vi "BackEnd_Module.vi"() -> ()   [LabVIEW 2023]
uses:
  Controls/Quantity_Data.ctl
  Controls/Queue_Operation_Select.ctl
  Controls/State_and_Data.ctl
  Controls/File_Operation_Select.ctl
panel:
  in  "Error_In":errorcluster
  out "error constant":errorcluster
  in  "Backend_Data":T1 {"Level"."Milk_Level" scale=0.0..100.0; "Level"."Bean_Level" scale=0.0..100.0; "Level"."Water_Level" scale=0.0..100.0}
  # "COFFEE MACHINE"
  # "Backend Control Panel"
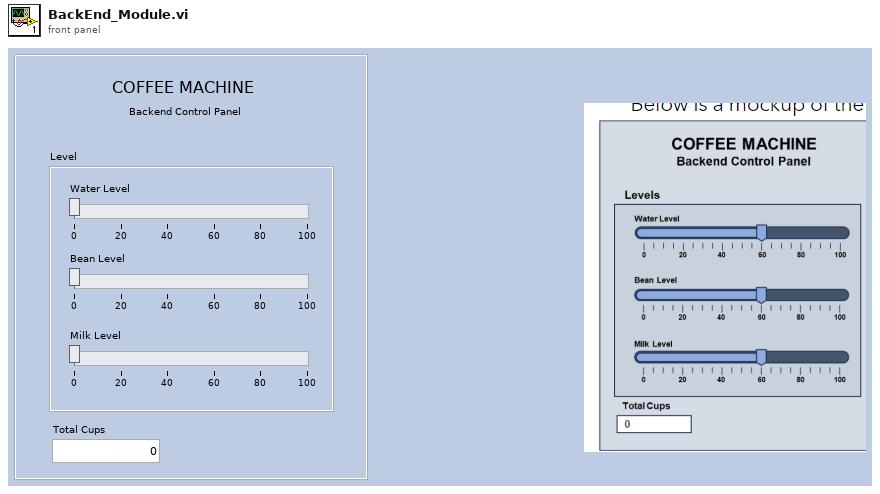
[diagram p1: front panel]
types:
  T1 = typedef "Quantity_Data.ctl" = cluster{"Level":cluster{"Water_Level":dbl, "Bean_Level":dbl, "Milk_Level":dbl}, "Total_Cups":dbl}
  T2 = typedef "File_Operation_Select.ctl" = enum16{"Open", "Read", "Write", "Close"}
  T3 = typedef "State_and_Data.ctl" = cluster{"State":string, "Data":variant}
  T4 = typedef "Queue_Operation_Select.ctl" = enum16{"Obtain_Queue", "Enqueue", "Enqueue_First", "Enqueue_N", "Lossy_Enqueue", "Preview", "Queue_Status", "Dequeue", "Flush", "Release_Queue"}
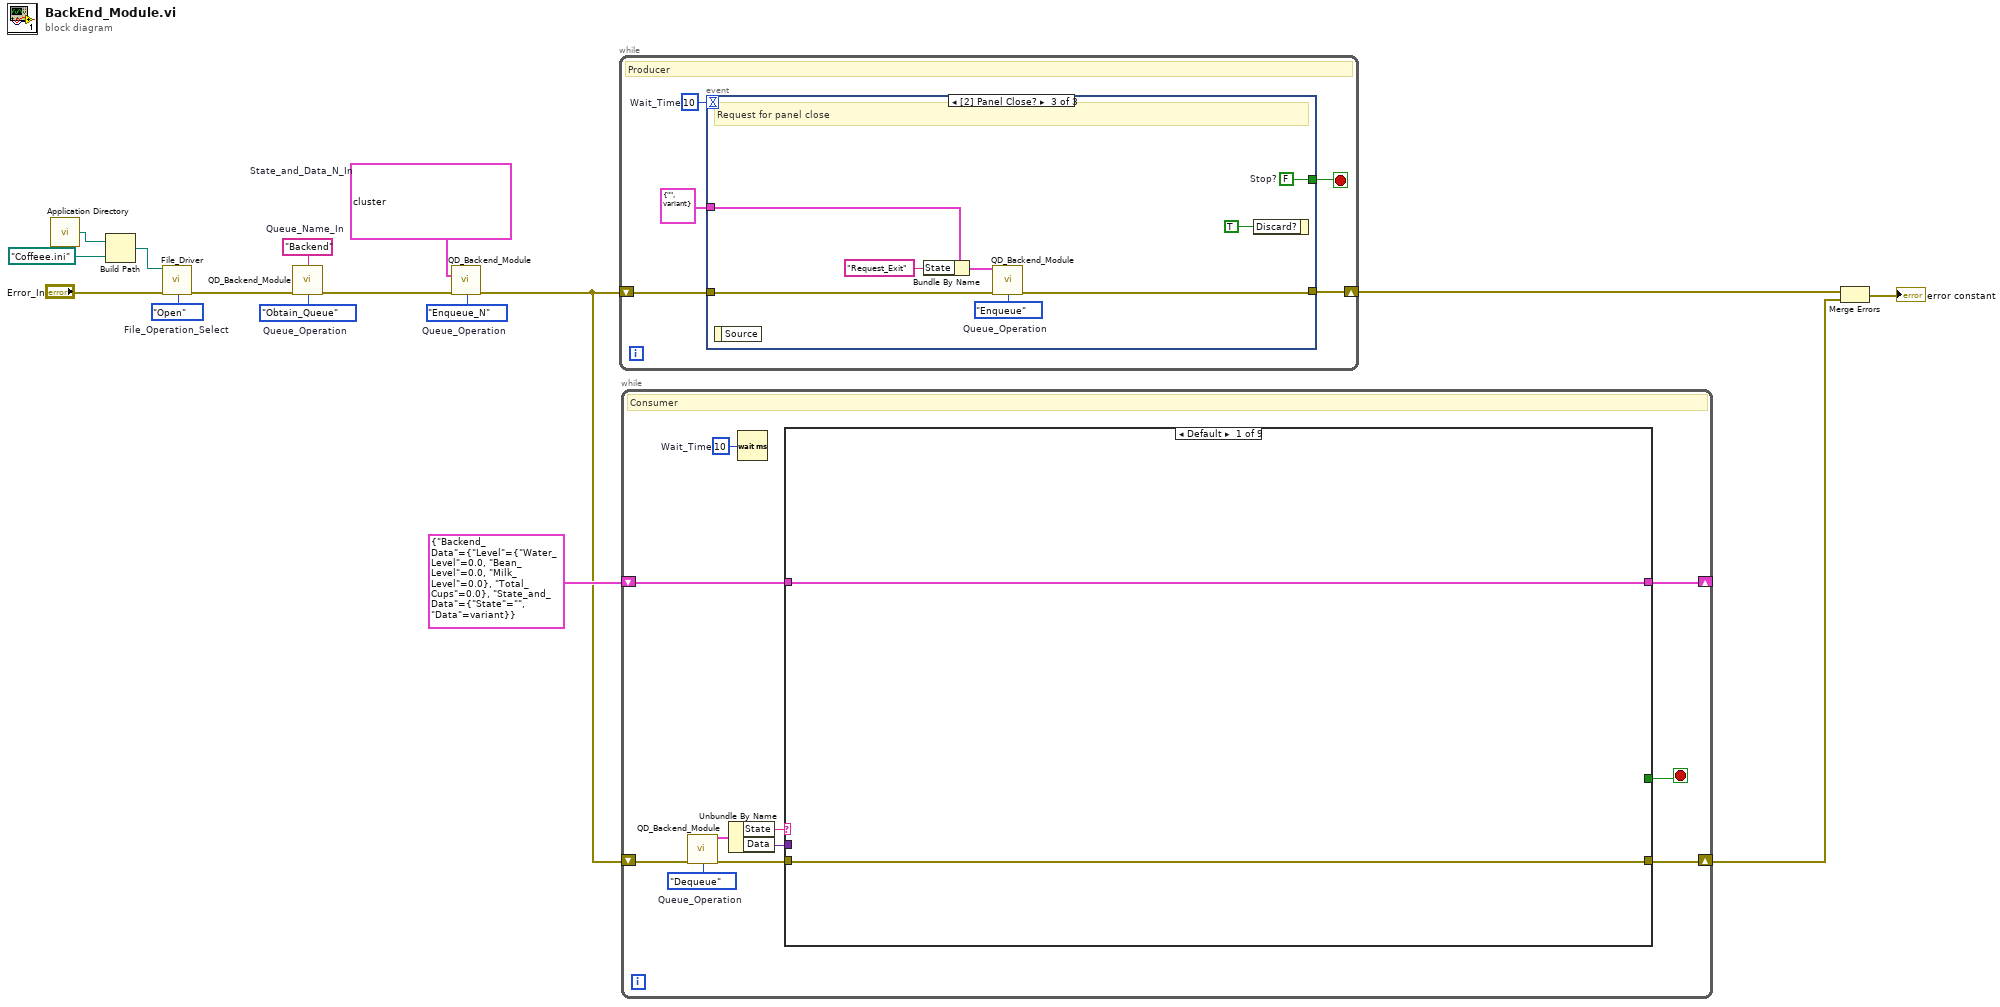
[diagram p0: block diagram]
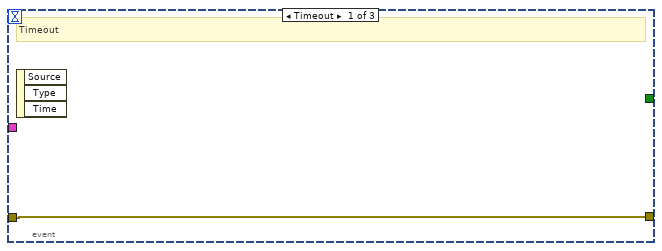
[diagram p2: hidden frame]
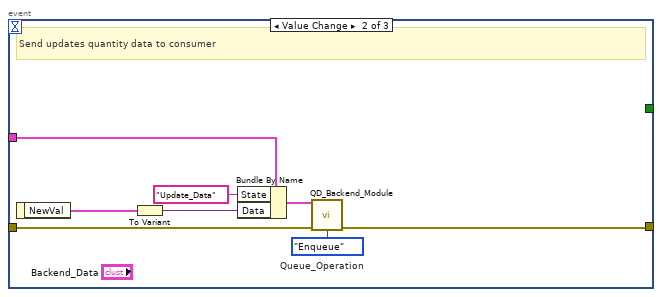
[diagram p3: hidden frame]
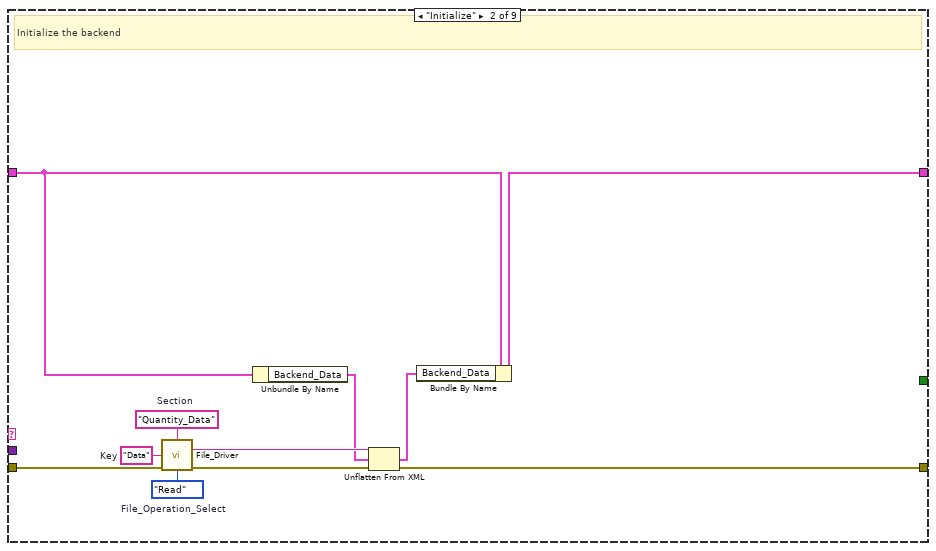
[diagram p4: hidden frame]
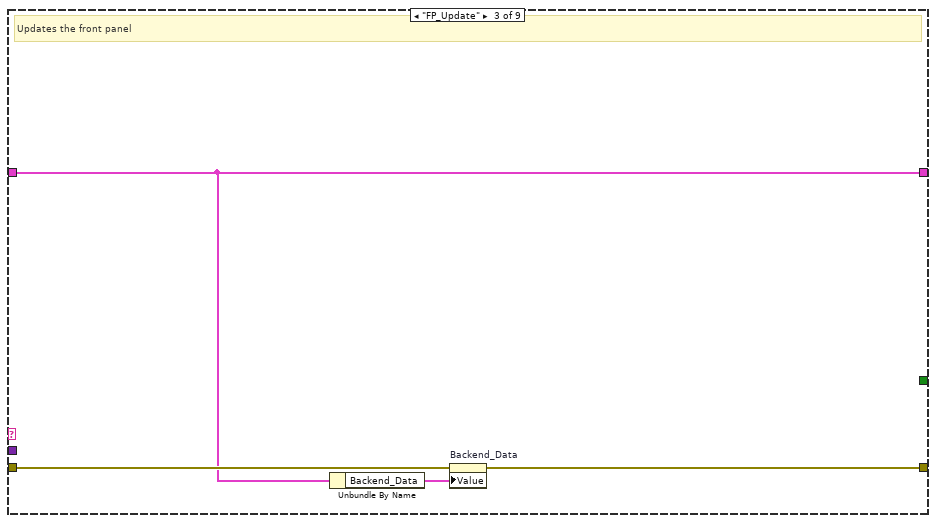
[diagram p5: hidden frame]
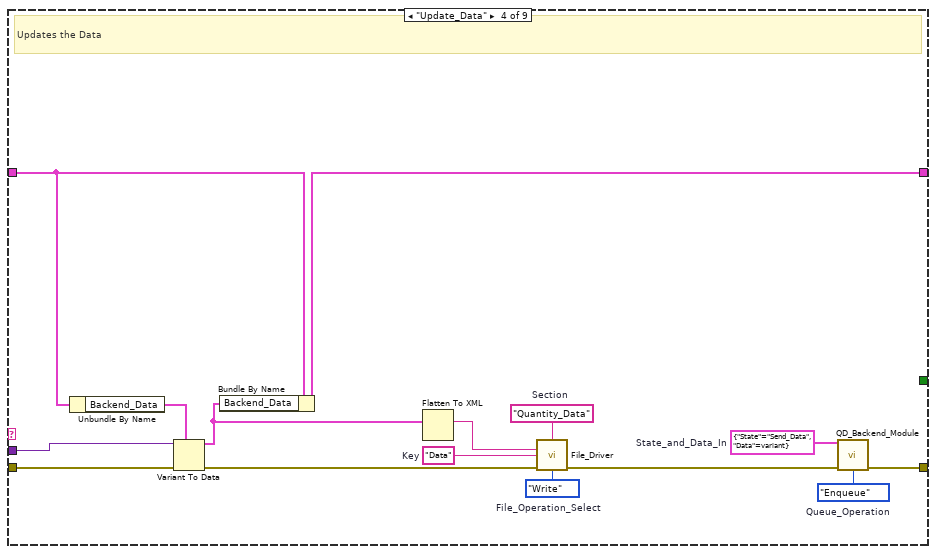
[diagram p6: hidden frame]
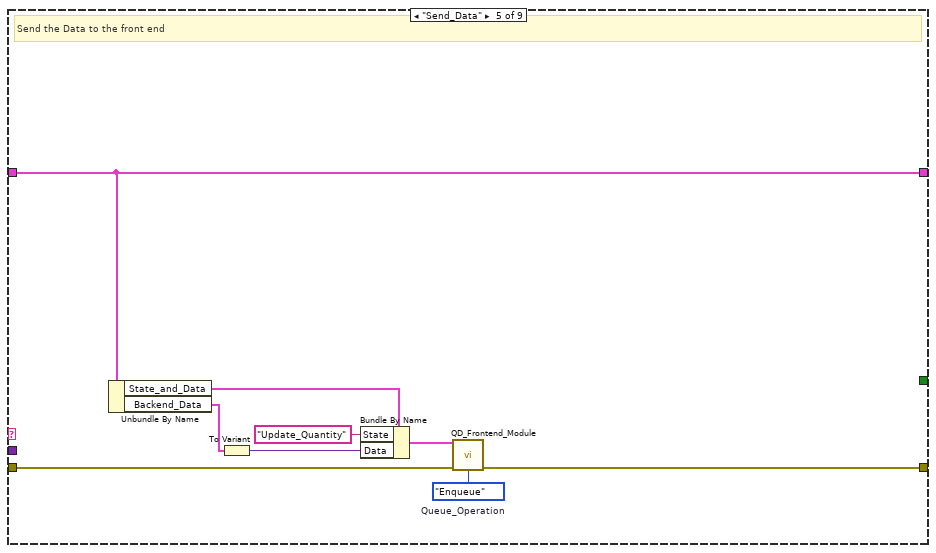
[diagram p7: hidden frame]
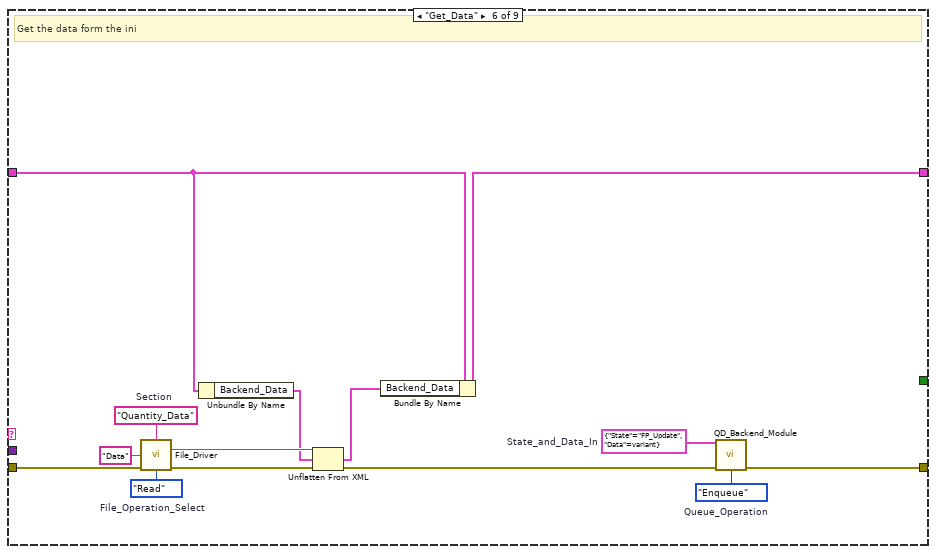
[diagram p8: hidden frame]
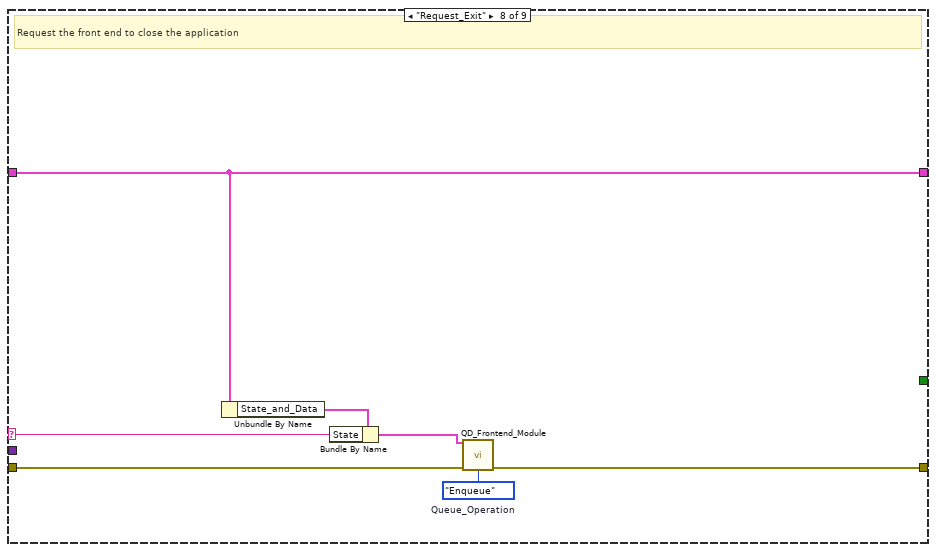
[diagram p10: hidden frame]
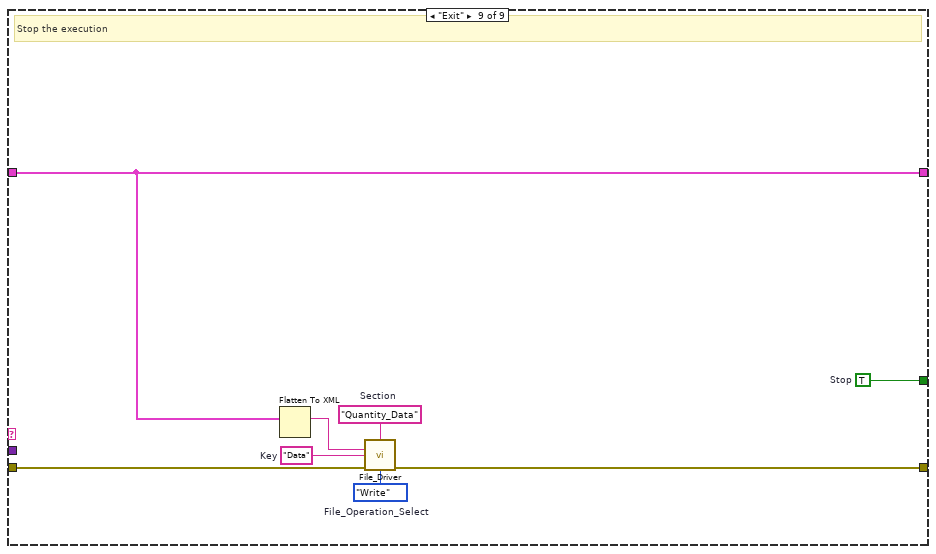
[diagram p11: hidden frame]
diagram:
  w5 = File_Operation_Select."Open"  # File_Operation_Select
  w10 = T3[] [{"State"="Initialize", "Data"=variant(cluster{"Current_Data":dbl, "Temp_Data":dbl} {"Current_Data"=0.0, "Temp_Data"=0.0})}, {"State"="FP_Update", "Data"=variant(cluster{"Current_Data":dbl, "Temp_Data":dbl} {"Current_Data"=0.0, "Temp_Data"=0.0})}]  # State_and_Data_N_In
  w11 = Queue_Operation_Select."Enqueue_N"  # Queue_Operation
  w12 = "Backend"  # Queue_Name_In
  w13 = Queue_Operation_Select."Obtain_Queue"  # Queue_Operation
  n1 = call <vilib>:"Application Directory.vi"() -> ("Application Directory"=w9:path)
  n2 = Build Path(base path=w9, name or relative path=path "Coffeee.ini") -> (appended path=w4:path)
  n3 = call "File_Driver.vi"("File_Path"=w4, "Error_In"="Error_In", "File_Operation_Select"=w5) -> ("Error_Out"=w6:errorcluster)  [unwired: 11 in, 1 out]
  n4 = call "QD_Backend_Module.vi"("Queue_Name_In"=w12, "Error_In"=w6, "Queue_Operation"=w13) -> ("Error_Out"=w14:errorcluster)  [unwired: 10 in, 2 out]
  n5 = call "QD_Backend_Module.vi"("State_and_Data_N_In"=w10, "Error_In"=w14, "Queue_Operation"=w11) -> ("Error_Out"=w1:errorcluster)  [unwired: 10 in, 2 out]
  n6 = while {
    shift-right: [w21] -> w16
    shift-left: w1 -> [w20]
    stop <- w19 stop-if-true
    w17 = 10  # Wait_Time
    # "Producer"
    n7 = event shown="[2] Panel Close?" {
      selector: _ -> [_ _ _]
      dyn-events: _ -> [_ _ _]
      timeout: w17 -> [_ _ _]
      tunnel: [w22 w29 w37] -> w21
      tunnel: w20 -> [w22 w30 w38]
      tunnel: [_ _ w34] -> w19
      tunnel: T3 {"State"="", "Data"=variant} ("State_and_Data_In") -> [_ w24 w32]
      event Timeout {
        # "Timeout"
        n8 = event-data() -> ()  [unwired: 1 in, 3 out]
      }
      event Value Change {
        w28 = Queue_Operation_Select."Enqueue"  # Queue_Operation
        # "Send updates quantity data to consumer"
        n9 = event-data() -> ("NewVal"=w26:T1)  [unwired: 1 in]
        n10 = To Variant(anything=w26) -> (Variant=w25:variant)
        n11 = Bundle By Name(cluster=w24, "State"="Update_Data", "Data"=w25) -> (w27:T3)
        n12 = call "QD_Backend_Module.vi"("State_and_Data_In"=w27, "Error_In"=w30, "Queue_Operation"=w28) -> ("Error_Out"=w29:errorcluster)  [unwired: 10 in, 2 out]
      }
      event Panel Close? {
        w34 = FALSE  # Stop?
        w36 = Queue_Operation_Select."Enqueue"  # Queue_Operation
        # "Request for panel close"
        n13 = event-data() -> ()  [unwired: 1 in, 1 out]
        n14 = Bundle By Name(cluster=w32, "State"="Request_Exit") -> (w35:T3)
        n15 = call "QD_Backend_Module.vi"("State_and_Data_In"=w35, "Error_In"=w38, "Queue_Operation"=w36) -> ("Error_Out"=w37:errorcluster)  [unwired: 10 in, 2 out]
        n16 = event-data("Discard?"=TRUE) -> ()  [unwired: 1 in, 1 out]
      }
    }
  }
  n17 = while {
    shift-right: [w49] -> w2
    shift-left: w1 -> [w48]
    shift-right: [w43] -> _
    shift-left: cluster{"Backend_Data":T1, "State_and_Data":T3} {"Backend_Data"={"Level"={"Water_Level"=0.0, "Bean_Level"=0.0, "Milk_Level"=0.0}, "Total_Cups"=0.0}, "State_and_Data"={"State"="", "Data"=variant}} -> [w42]
    stop <- w41 stop-if-true
    w40 = u32 10  # Wait_Time
    w46 = Queue_Operation_Select."Dequeue"  # Queue_Operation
    # "Consumer"
    n18 = call "QD_Backend_Module.vi"("Error_In"=w48, "Queue_Operation"=w46) -> ("State_and_Data_Out"=w39:T3, "Error_Out"=w47:errorcluster)  [unwired: 11 in, 1 out]
    n19 = Unbundle By Name(w39) -> ("State"=w45:string, "Data"=w44:variant)
    n20 = Wait (ms)(milliseconds to wait=w40) -> ()  [unwired: 1 out]
    n21 = case shown="Default" w45 {
      selector: w45 -> [_ _ _ _ _ _ _ w108 _]
      tunnel: [w51 w52 w65 w69 w89 w103 w106 w112 w120] -> w49
      tunnel: w47 -> [w51 w62 w66 w81 w90 w100 w106 w113 w121]
      tunnel: w44 -> [_ _ _ w78 _ _ _ _ _]
      tunnel: [w50 w54 w64 w80 w88 w104 w105 w110 w116] -> w43
      tunnel: w42 -> [w50 w56 w64 w77 w88 w92 w105 w110 w116]
      tunnel: [_ _ _ _ _ _ _ _ w114] -> w41
      frame Default {
      }
      frame "Initialize" {
        w58 = "Data"  # Key
        w59 = "Quantity_Data"  # Section
        w60 = File_Operation_Select."Read"  # File_Operation_Select
        # "Initialize the backend"
        n22 = call "File_Driver.vi"("Section"=w59, "Key"=w58, "Error_In"=w62, "File_Operation_Select"=w60) -> ("Data_Out"=w57:string, "Error_Out"=w61:errorcluster)  [unwired: 10 in]
        n23 = Unbundle By Name(w56) -> ("Backend_Data"=w55:T1)
        n24 = Unflatten From XML(xml string=w57, type=w55, error in (no error)=w61) -> (value=w53:T1, error out=w52:errorcluster)
        n25 = Bundle By Name(cluster=w56, "Backend_Data"=w53) -> (w54:cluster{"Backend_Data":T1, "State_and_Data":T3})
      }
      frame "FP_Update" {
        # "Updates the front panel"
        n26 = Unbundle By Name(w64) -> ("Backend_Data"=w63:T1)
        n27 = property on="Backend_Data" class="Clust (strict)"(error in=w66, "Value"=w63) -> (error out=w65:errorcluster)  [unwired: 1 in, 1 out]
      }
      frame "Update_Data" {
        w67 = Queue_Operation_Select."Enqueue"  # Queue_Operation
        w68 = T3 {"State"="Send_Data", "Data"=variant}  # State_and_Data_In
        w72 = "Quantity_Data"  # Section
        w73 = "Data"  # Key
        w74 = File_Operation_Select."Write"  # File_Operation_Select
        # "Updates the Data"
        n28 = Unbundle By Name(w77) -> ("Backend_Data"=w76:T1)
        n29 = Variant To Data(error in=w81, type=w76, Variant=w78) -> (data=w71:T1, error out=w79:errorcluster)
        n30 = Bundle By Name(cluster=w77, "Backend_Data"=w71) -> (w80:cluster{"Backend_Data":T1, "State_and_Data":T3})
        n31 = Flatten To XML(6:w71) -> (2:w70:string)
        n32 = call "File_Driver.vi"("Section"=w72, "Data_In"=w70, "Key"=w73, "Error_In"=w79, "File_Operation_Select"=w74) -> ("Error_Out"=w75:errorcluster)  [unwired: 9 in, 1 out]
        n33 = call "QD_Backend_Module.vi"("State_and_Data_In"=w68, "Error_In"=w75, "Queue_Operation"=w67) -> ("Error_Out"=w69:errorcluster)  [unwired: 10 in, 2 out]
      }
      frame "Send_Data" {
        w84 = Queue_Operation_Select."Enqueue"  # Queue_Operation
        # "Send the Data to the front end"
        n34 = Unbundle By Name(w88) -> ("State_and_Data"=w86:T3, "Backend_Data"=w83:T1)
        n35 = To Variant(anything=w83) -> (Variant=w82:variant)
        n36 = Bundle By Name(cluster=w86, "State"="Update_Quantity", "Data"=w82) -> (w87:T3)
        n37 = call "QD_Frontend_Module.vi"("State_and_Data_In"=w87, "Error_In"=w90, "Queue_Operation"=w84) -> ("Error_Out"=w89:errorcluster)  [unwired: 10 in, 2 out]
      }
      frame "Get_Data" {
        w97 = "Quantity_Data"  # Section
        w98 = File_Operation_Select."Read"  # File_Operation_Select
        w101 = T3 {"State"="FP_Update", "Data"=variant}  # State_and_Data_In
        w102 = Queue_Operation_Select."Enqueue"  # Queue_Operation
        # "Get the data form the ini"
        n38 = call "File_Driver.vi"("Section"=w97, "Key"="Data", "Error_In"=w100, "File_Operation_Select"=w98) -> ("Data_Out"=w93:string, "Error_Out"=w99:errorcluster)  [unwired: 10 in]
        n39 = Unbundle By Name(w92) -> ("Backend_Data"=w91:T1)
        n40 = Unflatten From XML(xml string=w93, type=w91, error in (no error)=w99) -> (value=w94:T1, error out=w95:errorcluster)
        n41 = Bundle By Name(cluster=w92, "Backend_Data"=w94) -> (w104:cluster{"Backend_Data":T1, "State_and_Data":T3})
        n42 = call "QD_Backend_Module.vi"("State_and_Data_In"=w101, "Error_In"=w95, "Queue_Operation"=w102) -> ("Error_Out"=w103:errorcluster)  [unwired: 10 in, 2 out]
      }
      frame "Error" {
        # "Handles  Error"
      }
      frame "Request_Exit" {
        w111 = Queue_Operation_Select."Enqueue"  # Queue_Operation
        # "Request the front end to close the application"
        n43 = Unbundle By Name(w110) -> ("State_and_Data"=w109:T3)
        n44 = Bundle By Name(cluster=w109, "State"=w108) -> (w107:T3)
        n45 = call "QD_Frontend_Module.vi"("State_and_Data_In"=w107, "Error_In"=w113, "Queue_Operation"=w111) -> ("Error_Out"=w112:errorcluster)  [unwired: 10 in, 2 out]
      }
      frame "Exit" {
        w114 = TRUE  # Stop
        w117 = "Data"  # Key
        w118 = "Quantity_Data"  # Section
        w119 = File_Operation_Select."Write"  # File_Operation_Select
        # "Stop the execution"
        n46 = Flatten To XML(6:w116) -> (2:w115:string)
        n47 = call "File_Driver.vi"("Section"=w118, "Data_In"=w115, "Key"=w117, "Error_In"=w121, "File_Operation_Select"=w119) -> ("Error_Out"=w120:errorcluster)  [unwired: 9 in, 1 out]
      }
    }
  }
  n48 = Merge Errors(w16, w2) -> (→"error constant":errorcluster)
